vi "initBothPDs.vi"(8 "error in (no error) 2":errorcluster caption="error in (no error)" {"code" format="%.0x"}, 9 "error in (no error)":errorcluster {"code" format="%.0x"}, 10 "resource name 2":refnum<visa-resource-name> caption="resource name", 11 "resource name":refnum<visa-resource-name>) -> (0 "error IO 2":errorcluster, 1 "error IO":errorcluster, 2 "instrument handle out 2":refnum<visa-resource-name> caption="instrument handle out", 3 "instrument handle out":refnum<visa-resource-name>, 5 "Initialized PD 2":bool, 7 "Initialized PD":bool)   [LabVIEW 2018]
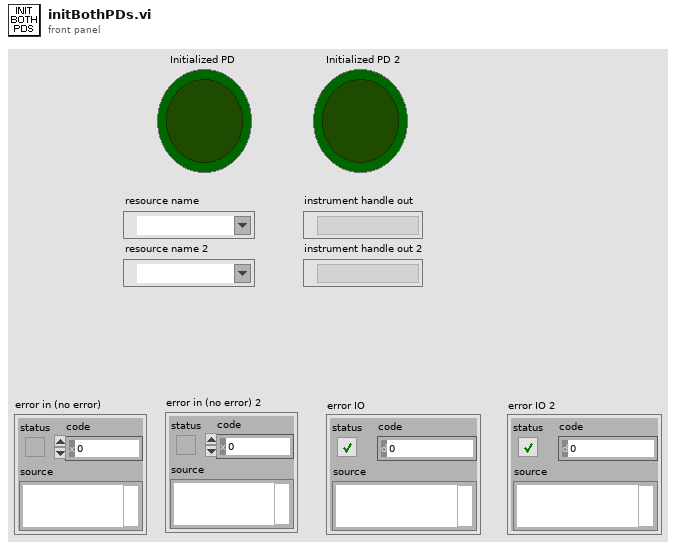
[diagram p1: front panel]
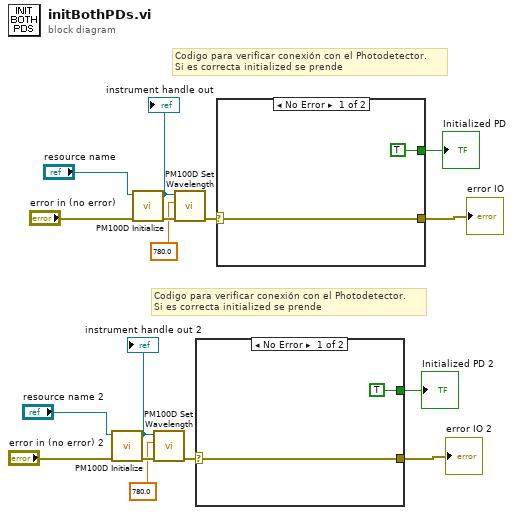
[diagram p0: block diagram]
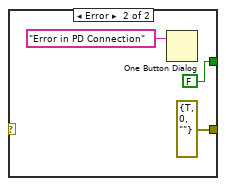
[diagram p2: hidden frame]
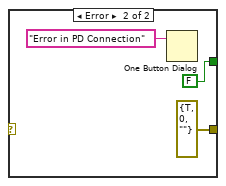
[diagram p3: hidden frame]
diagram:
  # "Codigo para verificar conexión con el Photodetector.\nSi es correcta initialized se prende"
  # "Codigo para verificar conexión con el Photodetector.\nSi es correcta initialized se prende"
  n1 = call "PM100D Initialize.vi"("error in (no error)"="error in (no error) 2", "resource name"="resource name 2") -> ("error out"=w5:errorcluster, "instrument handle out"=w6:refnum<visa-resource-name>)  [unwired: 8 in]
  "instrument handle out 2" <- w6
  n2 = call "PM100D Initialize.vi"("error in (no error)"="error in (no error)", "resource name"="resource name") -> ("error out"=w13:errorcluster, "instrument handle out"=w14:refnum<visa-resource-name>)  [unwired: 8 in]
  "instrument handle out" <- w14
  n3 = call "PM100D Set Wavelength.vi"("error in (no error)"=w5, "Wavelength (0.0)"=780.0, "instrument handle"=w6) -> ("error out"=w4:errorcluster)  [unwired: 7 in, 1 out]
  n4 = call "PM100D Set Wavelength.vi"("error in (no error)"=w13, "Wavelength (0.0)"=780.0, "instrument handle"=w14) -> ("error out"=w12:errorcluster)  [unwired: 7 in, 1 out]
  n5 = case shown="No Error" w4 {
    selector: w4 -> [w18 _]
    tunnel: [w18 errorcluster {"status"=TRUE, "code"=0, "source"=""} ("error IO")] -> w1
    tunnel: [TRUE FALSE ("Initialized PD")] -> w3
    frame No Error {
    }
    frame Error {
      n6 = One Button Dialog(message="Error in PD Connection") -> ()  [unwired: 1 in, 1 out]
    }
  }
  "Initialized PD 2" <- w3
  "error IO 2" <- w1
  n7 = case shown="No Error" w12 {
    selector: w12 -> [w23 _]
    tunnel: [w23 errorcluster {"status"=TRUE, "code"=0, "source"=""} ("error IO")] -> w9
    tunnel: [TRUE FALSE ("Initialized PD")] -> w11
    frame No Error {
    }
    frame Error {
      n8 = One Button Dialog(message="Error in PD Connection") -> ()  [unwired: 1 in, 1 out]
    }
  }
  "Initialized PD" <- w11
  "error IO" <- w9
